vi "setUp.vi"(8 "error in (no error)":errorcluster, 11 "TestITransportAPISemantics In":refnum<class "TestITransportAPISemantics.lvclass">) -> (0 "error out":errorcluster, 3 "TestITransportAPISemantics Out":refnum<class "TestITransportAPISemantics.lvclass">)   [LabVIEW 2017, in "TestITransportAPISemantics.lvclass"]
doc: "setUp runs prior to the test method during test execution. Use this method to initialize any object data required by your tests."
uses:
  TestITransportAPISemantics.lvclass
  C:/Program Files (x86)/National Instruments/LabVIEW 2017/vi.lib/addons/_JKI Toolkits/VI Tester/TestCase.llb/TestCase.lvclass
  Source/Concrete/BooleanTextBinding/BooleanTextBinding.lvclass
  C:/Git/composed-transport/Source/ITransport/ITransport.lvclass
  Source/Concrete/ConfigurationFileBinding/ConfigurationFileBinding.lvclass
  Source/Concrete/EventTransport/EventTransport.lvclass
  Source/Concrete/FormattedStringBinding/FormattedStringBinding.lvclass
  Source/Concrete/ListboxItemNamesBinding/ListboxItemNamesBinding.lvclass
  Source/Concrete/MCListboxItemNamesBinding/MCListboxItemNamesBinding.lvclass
  Source/Concrete/NotifierTransport/NotifierTransport.lvclass
  Source/Concrete/PersistToDiskTransport/PersistToDiskTransport.lvclass
  Source/Concrete/QueueTransport/QueueTransport.lvclass
  Source/Concrete/RingStringsBinding/RingStringsBinding.lvclass
  Source/Concrete/StreamToDiskTransport/StreamToDiskTransport.lvclass
  Source/Concrete/TerminalCaptionBinding/TerminalCaptionBinding.lvclass
  Source/Concrete/TerminalEnabledStateBinding/TerminalEnabledStateBinding.lvclass
  Source/Concrete/TerminalPropertyBinding/TerminalPropertyBinding.lvclass
  Source/Concrete/TerminalSignalingValueBinding/TerminalSignalingValueBinding.lvclass
  Source/Concrete/TerminalValueBinding/TerminalValueBinding.lvclass
  Source/Concrete/TerminalVisibilityBinding/TerminalVisibilityBinding.lvclass
  Source/Concrete/ValueReferenceTransport/ValueReferenceTransport.lvclass
  Source/Concrete/ActorMessageTransport/ActorMessageTransport.lvclass
  TestITransportAPISemantics.lvclass/TestITransportAPISemantics.ctl
  <vilib>/addons/_JKI Toolkits/VI Tester/TestCase.llb/TestCase.lvclass
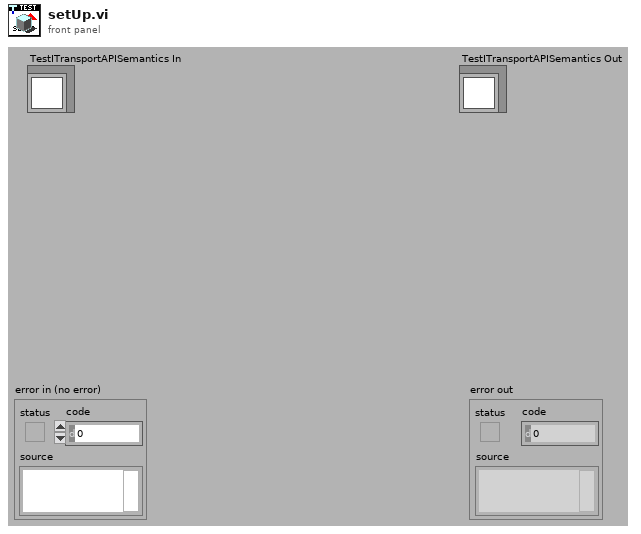
[diagram p1: front panel]
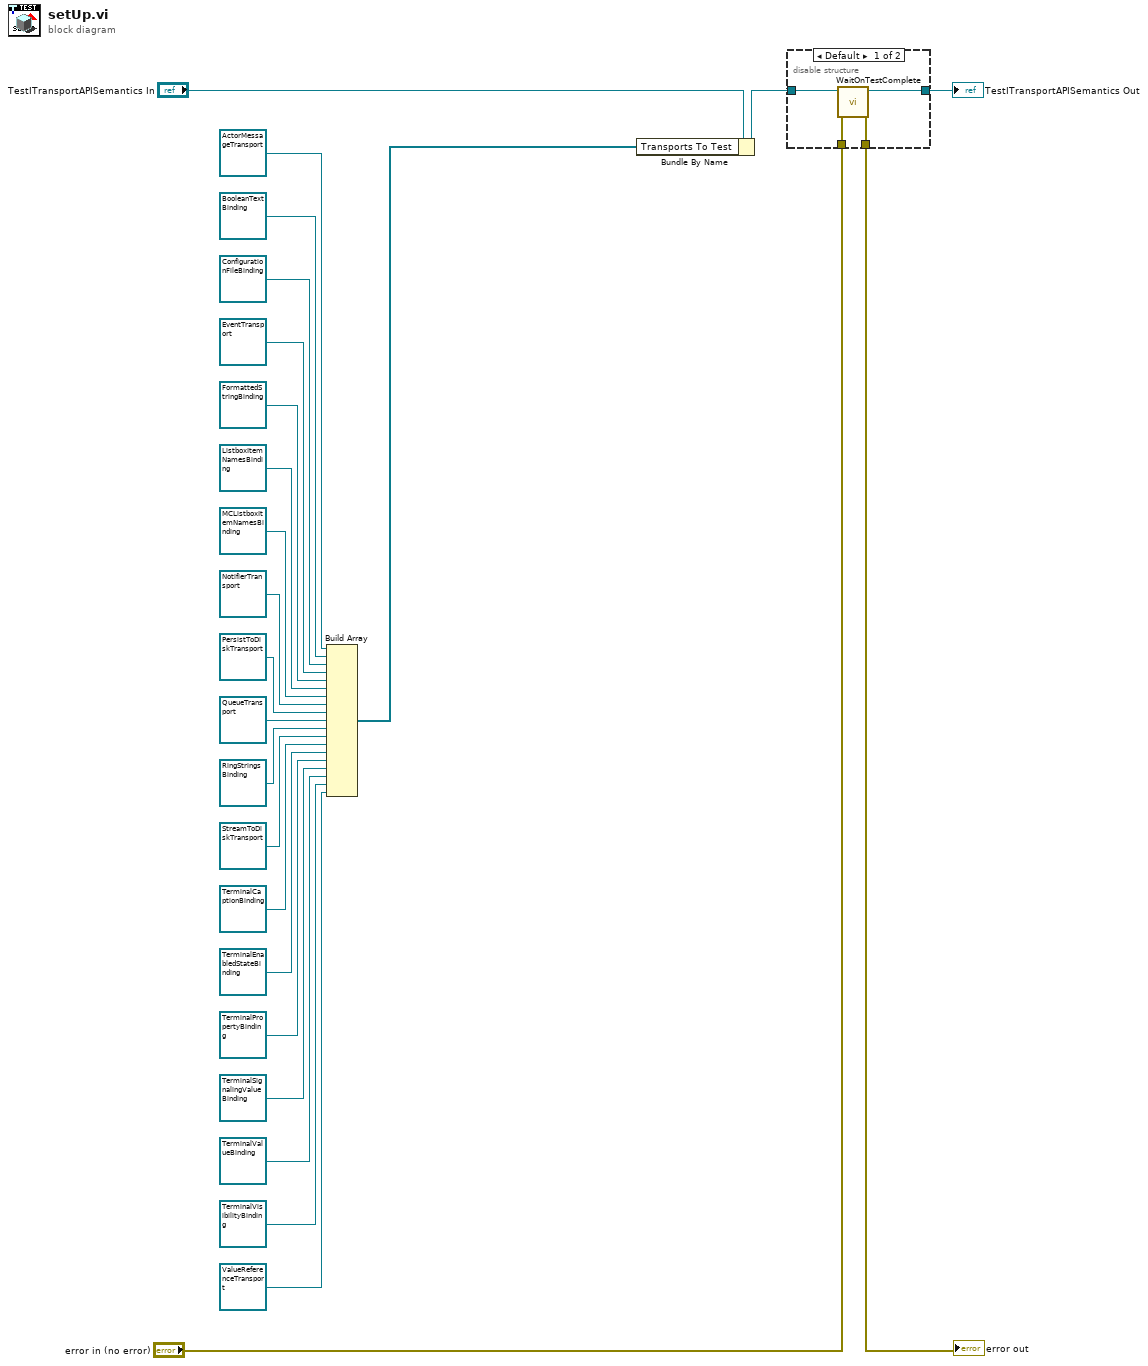
[diagram p0: block diagram]
diagram:
  n1 = Build Array(refnum<class "ActorMessageTransport.lvclass"> refnum ("ActorMessageTransport.lvlib:ActorMessageTransport.lvclass"), refnum<class "BooleanTextBinding.lvclass"> refnum ("BooleanTextBinding.lvclass"), refnum<class "ConfigurationFileBinding.lvclass"> refnum ("ConfigurationFileBinding.lvclass"), refnum<class "EventTransport.lvclass"> refnum ("EventTransport.lvclass"), refnum<class "FormattedStringBinding.lvclass"> refnum ("FormattedStringBinding.lvclass"), refnum<class "ListboxItemNamesBinding.lvclass"> refnum ("ListboxItemNamesBinding.lvclass"), refnum<class "MCListboxItemNamesBinding.lvclass"> refnum ("MCListboxItemNamesBinding.lvclass"), refnum<class "NotifierTransport.lvclass"> refnum ("NotifierTransport.lvclass"), refnum<class "PersistToDiskTransport.lvclass"> refnum ("PersistToDiskTransport.lvclass"), refnum<class "QueueTransport.lvclass"> refnum ("QueueTransport.lvclass"), refnum<class "RingStringsBinding.lvclass"> refnum ("RingStringsBinding.lvclass"), refnum<class "StreamToDiskTransport.lvclass"> refnum ("StreamToDiskTransport.lvclass"), refnum<class "TerminalCaptionBinding.lvclass"> refnum ("TerminalCaptionBinding.lvclass"), refnum<class "TerminalEnabledStateBinding.lvclass"> refnum ("TerminalEnabledStateBinding.lvclass"), refnum<class "TerminalPropertyBinding.lvclass"> refnum ("TerminalPropertyBinding.lvclass"), refnum<class "TerminalSignalingValueBinding.lvclass"> refnum ("TerminalSignalingValueBinding.lvclass"), refnum<class "TerminalValueBinding.lvclass"> refnum ("TerminalValueBinding.lvclass"), refnum<class "TerminalVisibilityBinding.lvclass"> refnum ("TerminalVisibilityBinding.lvclass"), refnum<class "ValueReferenceTransport.lvclass"> refnum ("ValueReferenceTransport.lvclass")) -> (w1:refnum<class "ITransport.lvclass">[])
  n2 = Bundle By Name(cluster="TestITransportAPISemantics In", "Transports To Test"=w1) -> (w21:refnum<class "TestITransportAPISemantics.lvclass">)
  n3 = disable-structure shown="Default" {
    disable-tunnel: "error in (no error)" -> [w29 w30]
    disable-tunnel: [w28 w30] -> w24
    disable-tunnel: [w27 w31] -> w23
    disable-tunnel: w21 -> [w26 w31]
    frame condition #0 (active) {
      n4 = call <vilib>:"WaitOnTestComplete.vi"("error in (no error)"=w29, "TestCase in"=w26) -> ("error out"=w28:errorcluster, "TestCase out"=w27:refnum<class "TestITransportAPISemantics.lvclass">)  [unwired: 8 in]
    }
    frame condition #1 {
    }
  }
  "error out" <- w24
  "TestITransportAPISemantics Out" <- w23
